vi "Open_Instr.vi"(8 "error in (no error)":errorcluster caption="entrée d'erreur (pas d'erreur)", 11 "Class Multimeter Multimeter en entrée":refnum<class "Class Instrument Spectrum_Analyser.lvclass">) -> (0 "error out":errorcluster caption="sortie d'erreur", 3 "Class Multimeter Multimeter en sortie":refnum<class "Class Instrument Spectrum_Analyser.lvclass">)   [LabVIEW 2020, in "Library Instrument & Equipement.lvlib" / "Library Instruments.lvlib" / "Class Instrument Spectrum_Analyser.lvclass"]
uses:
  Class Instrument Spectrum_Analyser.lvclass
  Class Instrument Spectrum_Analyser.lvclass/Class Instrument Spectrum_Analyser.ctl
  Instrument (Default)/Class Instrument (Default).lvclass
  Spectrum Analyser/Class Spectrum Analyser (Default)/Class Spectrum Analyser (Default).lvclass
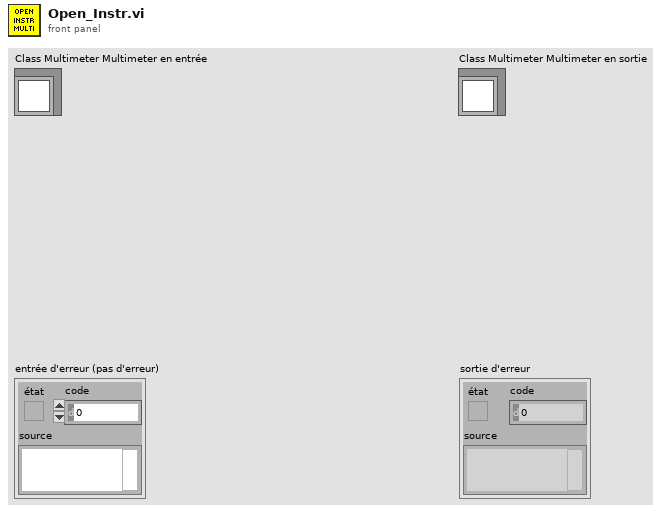
[diagram p1: front panel]
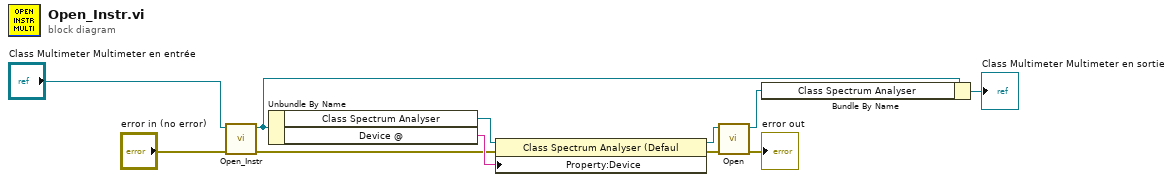
[diagram p0: block diagram]
diagram:
  n1 = call-parent "Open_Instr.vi"("error in (no error)"="error in (no error)", "Class Multimeter (Default) en entrée"="Class Multimeter Multimeter en entrée") -> ("error out"=w1:errorcluster, "Class Multimeter (Default) en sortie"=w8:refnum<class "Class Instrument Spectrum_Analyser.lvclass">)  [unwired: 8 in]
  n2 = Unbundle By Name(w8) -> ("Class Spectrum Analyser"=w2:refnum<class "Class Spectrum Analyser (Default).lvclass">, "Device @"=w3:string)
  n3 = property class="Class Spectrum Analyser (Defaul"(reference=w2, error in=w1, "Property:Device"=w3) -> (reference out=w5:refnum<class "Class Spectrum Analyser (Default).lvclass">, error out=w7:errorcluster)
  n4 = call-dynamic "Open.vi"("error in (no error)"=w7, "Class Spectrum Analyser (Default) en entrée"=w5) -> ("error out"=→"error out":errorcluster, "Class Spectrum Analyser (Default) en sortie"=w4:refnum<class "Class Spectrum Analyser (Default).lvclass">)  [unwired: 8 in]
  n5 = Bundle By Name(cluster=w8, "Class Spectrum Analyser"=w4) -> (→"Class Multimeter Multimeter en sortie":refnum<class "Class Instrument Spectrum_Analyser.lvclass">)
